vi "Initialize 1553 Driver.vi"(8 "Error in":errorcluster) -> (0 "Error out":errorcluster)   [LabVIEW 2020, in "AIM MIL-STD-1553 Hardware API.lvlib"]
uses:
  AIM MIL-STD-1553 Hardware API.lvlib
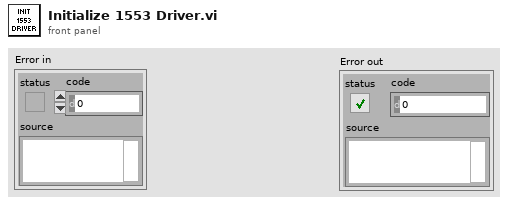
[diagram p1: front panel]
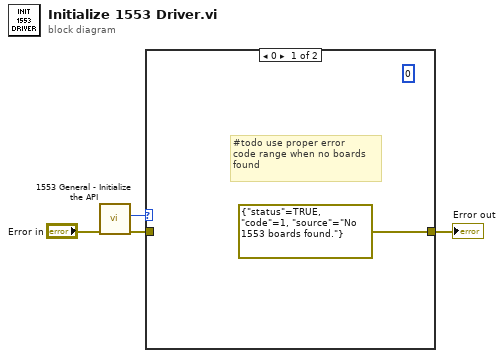
[diagram p0: block diagram]
diagram:
  n1 = call <instrlib>:"1553 General - Initialize the API.vi"("Error In (none)"="Error in") -> ("Error Out"=w4:errorcluster, "Modules Found"=w3:i32)  [unwired: 9 in]
  n2 = case shown="0" w3 {
    tunnel: w4 -> [_ w6]
    tunnel: [errorcluster {"status"=TRUE, "code"=1, "source"="No 1553 boards found."} ("Error Out") w6] -> w1
    frame 0 {
      (unwired) u32 0 ("Module Handle")
      # "#todo use proper error\ncode range when no boards\nfound"
    }
    frame Default {
    }
  }
  "Error out" <- w1
